vi "XY Scanning with Alazar.vi"() -> ()   [LabVIEW 2018]
uses:
  General/Controls/System Parameters.ctl
  General/Controls/Optical Parameters.ctl
  General/Controls/Vibratome Parameters.ctl
  General/Controls/Translation Stage Parameters.ctl
  Hardware Mfg/Thorlabs Translation Stages/Controls/Translation Stage Cluster.ctl
  General/Controls/Translation Stage Types.ctl
  General/Controls/Imaging Parameters.ctl
  General/Controls/Scan Direction.ctl
  Hardware Mfg/AlazarTech SDK/Controls/Clock Controls.ctl
  Hardware Mfg/AlazarTech SDK/Controls/Alazar Device ID.ctl
  Hardware Mfg/AlazarTech SDK/Controls/Channel Input Controls.ctl
  Hardware Mfg/AlazarTech SDK/Controls/General Trigger Settings.ctl
  Hardware Mfg/AlazarTech SDK/Controls/Trigger Engine Controls.ctl
  Hardware Mfg/AlazarTech SDK/Controls/Alazar Acquisition Settings.ctl
  General/actions/file type.ctl
  Hardware Mfg/AlazarTech SDK/Controls/Alazar Engine Actions.ctl
  General/Queue Manager Actions.ctl
  General/data manager action.ctl
  <vilib>/ErrorRing/Error Ring.xnode
panel:
  in  "file (use dialog)":path
  in  "File Type":T1
  in  "data action":enum16{"display", "save"}(ring)
  out "visulization time":dbl
  out "buffer enqueue time":dbl
  out "Image":T2(plugin-control)
  out "error out":errorcluster
  in  "stop":bool
  in  "Acq Settings":T3={"Window Type"=1, "Record Length"=1440, "Footer"=0, "Output Format"=11, "Offset"=0, "Records Per Buffer"=2048, "Records Count (Records/Acq)"=2147483647} {"Window Type" items=["DSP_WINDOW_NONE", "DSP_WINDOW_HANNING", "DSP_WINDOW_HAMMING", "DSP_WINDOW_BLACKMAN", "DSP_WINDOW_BLACKMAN_HARRIS", "DSP_WINDOW_BARTLETT"]; "Footer" items=["FOOTER_NONE", "FOOTER_NPT"]; "Output Format" items=["FLOAT_AMP2"=10, "FLOAT_LOG"=11]}
  in  "Trigger Settings":T6={"General Trigger Settings"={"Trigger Operation"=0, "Coupling ID"=2, "Range ID"=2, "Delay"=0, "Timeout Ticks"=0, "Mode"=0, "Parameter"=0}, "Trigger Engine 1"={"Trigger Engine"=0, "Source"=2, "Slope"=1, "Level"=140}, "Trigger Engine 2"={"Trigger Engine"=1, "Source"=3, "Slope"=1, "Level"=140}} {"General Trigger Settings"."Trigger Operation" items=["J", "K", "J OR K", "J AND K", "J XOR K", "J AND NOT K", "NOT J AND K"]; "General Trigger Settings"."Coupling ID" items=["AC"=1, "DC"=2]; "General Trigger Settings"."Range ID" items=["5 V", "1 V", "TTL"]; "Trigger Engine 1"."Trigger Engine" items=["J", "K"]; "Trigger Engine 1"."Source" items=["A", "B", "External", "Disable", "C", "D"]; "Trigger Engine 1"."Slope" items=["Positive"=1, "Negative"=2]; "Trigger Engine 2"."Trigger Engine" items=["J", "K"]; "Trigger Engine 2"."Source" items=["A", "B", "External", "Disable", "C", "D"]; "Trigger Engine 2"."Slope" items=["Positive"=1, "Negative"=2]}
  in  "Ch B Input Control":T7={"Channel"=2, "Coupling"=2, "Range"=10, "Impedance"=2} {"Channel" items=["A"=1, "B"=2, "C"=4, "D"=8]; "Coupling" items=["AC"=1, "DC"=2]; "Range" items=["20 mV"=1, "40 mV"=2, "50 mV"=3, "80 mV"=4, "100 mV"=5, "200 mV"=6, "400 mV"=7, "500 mV"=8, "800 mV"=9, "1 V"=10, "1.25 V"=33, "2 V"=11, "4 V"=12, "5 V"=13, "8 V"=14, "10 V"=15, "20 V"=16]; "Impedance" items=["1 MOhm"=1, "50 Ohm"=2, ""=0]}
  in  "Ch A Input Control":T7={"Channel"=1, "Coupling"=2, "Range"=10, "Impedance"=2} {"Channel" items=["A"=1, "B"=2, "C"=4, "D"=8]; "Coupling" items=["AC"=1, "DC"=2]; "Range" items=["20 mV"=1, "40 mV"=2, "50 mV"=3, "80 mV"=4, "100 mV"=5, "200 mV"=6, "400 mV"=7, "500 mV"=8, "800 mV"=9, "1 V"=10, "1.25 V"=33, "2 V"=11, "4 V"=12, "5 V"=13, "8 V"=14, "10 V"=15, "20 V"=16]; "Impedance" items=["1 MOhm"=1, "50 Ohm"=2, ""=0]}
  in  "Device ID":T8={"System ID"=1, "Board ID"=1}
  in  "Capture Clock":T9={"Sample Rate"=100, "Decimation"=0, "Source"=2, "Edge"=0} {"Edge" items=["Rising", "Falling"]; "Source" items=["Internal"=1, "Fast External"=2, "Medium External"=3, "Slow External"=4, "External AC"=5, "External DC"=6, "External 10MHz"=7]}
  in  "System Parameters":T10={"Optical Parameters"={"Obj. Focal Length [mm]"=45.0, "Scan Lens EFL[mm]"=60.0, "Tube Lens EFL[mm]"=180.0, "Galvo V Range (+/-)"=10.0, "Galvo Max Half Angle [Deg]"=19.0, "Max Galvo Range[%]"=0.0}, "Vibratome"={"Z Bottom [mm]"=0.0, "Pre Cut Dwell [s]"=0.0, "Blade Frequency [RPM]"=0, "Slice Speed [mm/s]"=0.0, "Post Cut Dwell [s]"=0.0, "Ramp Time [s]"=0.0, "Start X [mm]"=0.0, "Start Y [mm]"=0.0, "Slice Length [mm]"=0.0, "Slice Axis"=enum."Y Axis", "Controller VISA Ref"="COM4"}, "Table Stages"={"X Stage"={"Position"=0.0, "Is.Enabled?"=FALSE, "Is.Connected?"=FALSE, "Device SN"="45876539", "AccelerationMaximum"=0.0, "VelocityMaximum"=0.0, "Acceleration"=0.0, "Velocity"=0.0, "waitTimeout (ms)"=0, "Model"=enum."None", "Is.Homed?"=FALSE}, "Y Stage"={"Position"=0.0, "Is.Enabled?"=FALSE, "Is.Connected?"=FALSE, "Device SN"="45876539", "AccelerationMaximum"=0.0, "VelocityMaximum"=0.0, "Acceleration"=0.0, "Velocity"=0.0, "waitTimeout (ms)"=0, "Model"=enum."None", "Is.Homed?"=FALSE}, "Z Stage"={"Position"=0.0, "Is.Enabled?"=FALSE, "Is.Connected?"=FALSE, "Device SN"="45876539", "AccelerationMaximum"=0.0, "VelocityMaximum"=0.0, "Acceleration"=0.0, "Velocity"=0.0, "waitTimeout (ms)"=0, "Model"=enum."None", "Is.Homed?"=FALSE}}, "Imaging Parameter"={"Raster Scan Direction"=enum."Uni Directional", "Pixel Dwell Time [Clock Cycles]"=1, "Flyback Time [Clock Cycles]"=150, "XY Center [um]"={"X"=1.0, "Y"=1.0}, "Pixel Step Size [um]"=4.0, "XY Image Size"=enum."2048 x 2048", "Custom"=FALSE, "Custom Size"={"X"=10, "Y"=10}, "Line Averages"=1}} {"Imaging Parameter"."Line Averages" min=1 max=30 step=1; "Imaging Parameter"."Flyback Time [Clock Cycles]" max=1000 step=1; "Imaging Parameter"."Pixel Step Size [um]" min=0.0 max=10.0 step=0.01; "Imaging Parameter"."Custom Size"."Y" min=1 max=30 step=1; "Imaging Parameter"."Custom Size"."X" min=1 max=30 step=1; "Imaging Parameter"."XY Center [um]"."Y" min=1.0 max=30.0 step=1.0; "Imaging Parameter"."XY Center [um]"."X" min=1.0 max=30.0 step=1.0; "Imaging Parameter"."Pixel Dwell Time [Clock Cycles]" max=10 step=1}
  in  "Galvo HW Parameters":T18={"Analog Out Channel"="GalvoCtrl/ao0,GalvoCtrl/ao1", "Min Voltage"=-10.0, "Max Voltage"=10.0, "Pixel Clock Source"="/GalvoCtrl/PFI0", "Sample Rate"=1000.0, "Line Clock Out Ch"="GalvoCtrl/port0/line0"}
  # "X"
  # "X"
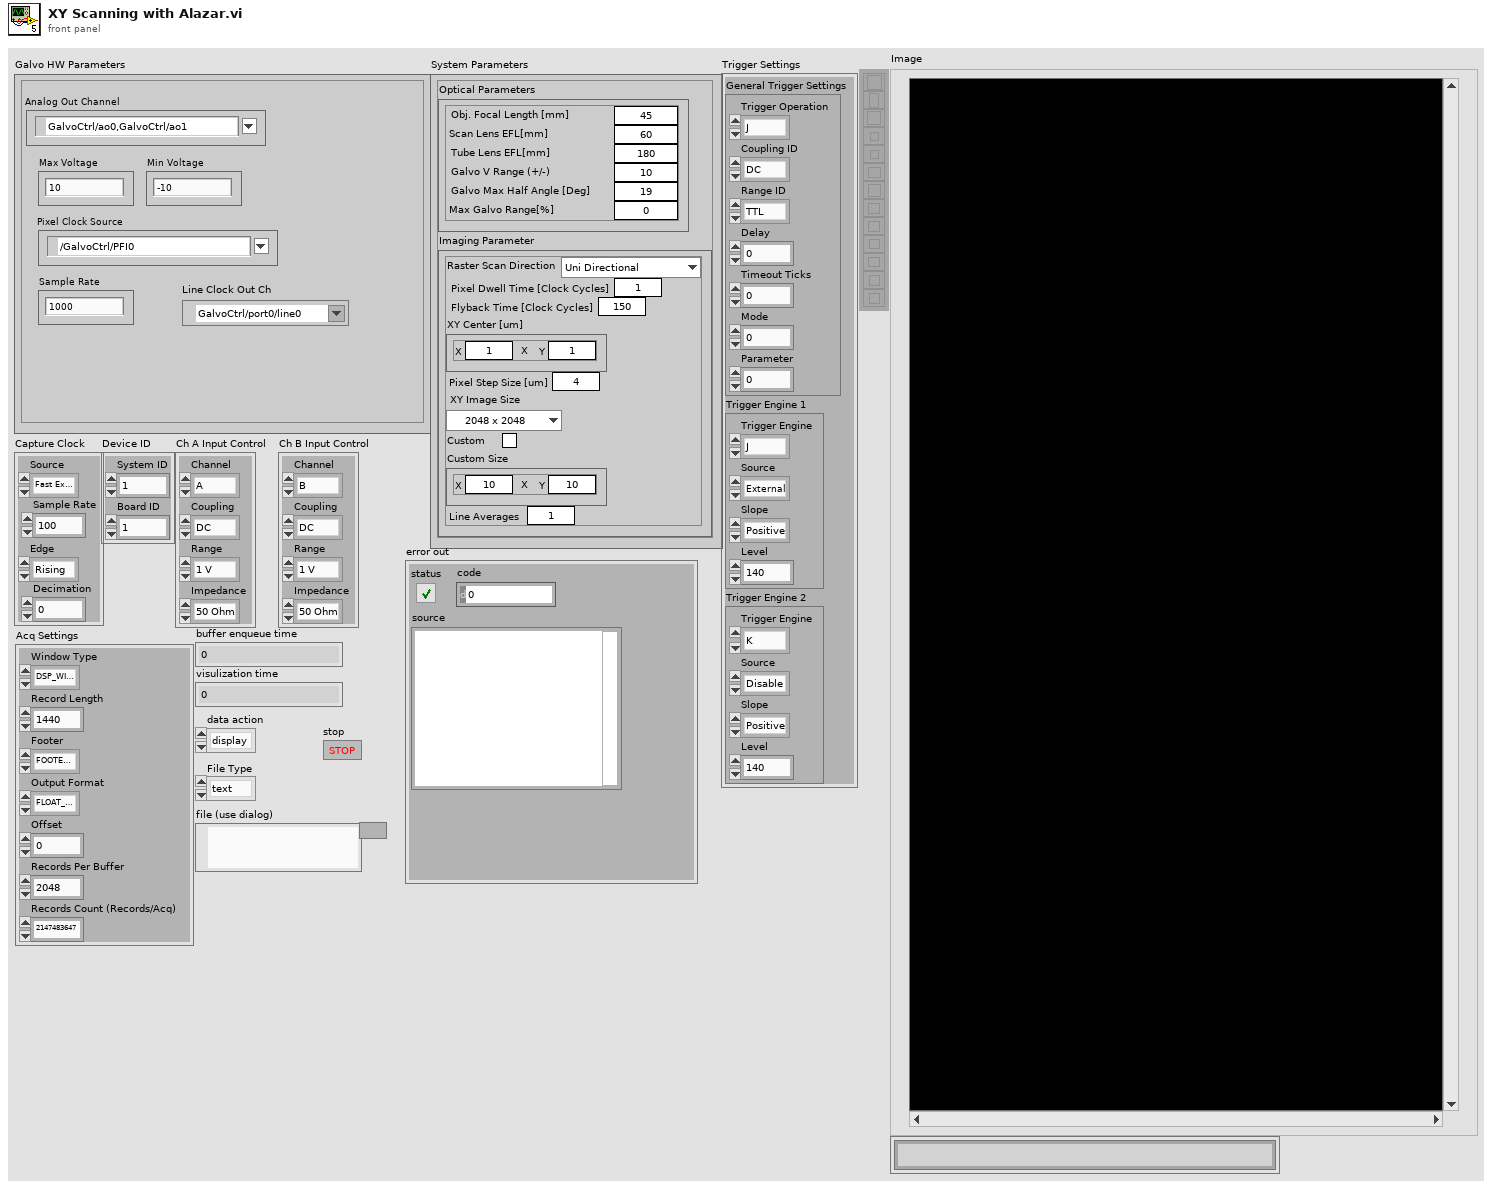
[diagram p1: front panel]
types:
  T1 = typedef "file type.ctl" = enum16{"text", "image", "binary"}
  T2 = typedef "IMAQ Image.ctl" = refnum<image>
  T3 = typedef "Alazar Acquisition Settings.ctl" = cluster{"Window Type":u32, "Record Length":u32, "Footer":u32, "Output Format":u32, "Offset":u32, "Records Per Buffer":u32, "Records Count (Records/Acq)":u32}
  T4 = typedef "General Trigger Settings.ctl" = cluster{"Trigger Operation":u32, "Coupling ID":u32, "Range ID":u32, "Delay":u32, "Timeout Ticks":u32, "Mode":u32, "Parameter":u32}
  T5 = typedef "Trigger Engine Controls.ctl" = cluster{"Trigger Engine":u32, "Source":u32, "Slope":u32, "Level":u32}
  T6 = cluster{"General Trigger Settings":T4, "Trigger Engine 1":T5, "Trigger Engine 2":T5}
  T7 = typedef "Channel Input Controls.ctl" = cluster{"Channel":u8, "Coupling":u32, "Range":u32, "Impedance":u32}
  T8 = typedef "Alazar Device ID.ctl" = cluster{"System ID":u32, "Board ID":u32}
  T9 = typedef "Clock Controls.ctl" = cluster{"Sample Rate":u32, "Decimation":u32, "Source":u32, "Edge":u32}
  T10 = typedef "System Parameters.ctl" = cluster{"Optical Parameters":T11, "Vibratome":T12, "Table Stages":T13, "Imaging Parameter":T16}
  T11 = typedef "Optical Parameters.ctl" = cluster{"Obj. Focal Length [mm]":dbl, "Scan Lens EFL[mm]":dbl, "Tube Lens EFL[mm]":dbl, "Galvo V Range (+/-)":dbl, "Galvo Max Half Angle [Deg]":dbl, "Max Galvo Range[%]":dbl}
  T12 = typedef "Vibratome Parameters.ctl" = cluster{"Z Bottom [mm]":dbl, "Pre Cut Dwell [s]":dbl, "Blade Frequency [RPM]":u16, "Slice Speed [mm/s]":dbl, "Post Cut Dwell [s]":dbl, "Ramp Time [s]":dbl, "Start X [mm]":dbl, "Start Y [mm]":dbl, "Slice Length [mm]":dbl, "Slice Axis":enum16{"X Axis", "Y Axis", "Z Axis"}, "Controller VISA Ref":refnum<visa-resource-name>}
  T13 = typedef "Translation Stage Parameters.ctl" = cluster{"X Stage":T14, "Y Stage":T14, "Z Stage":T14}
  T14 = typedef "Translation Stage Cluster.ctl" = cluster{"Position":dbl, "Is.Enabled?":bool, "Is.Connected?":bool, "Device SN":string, "AccelerationMaximum":dbl, "VelocityMaximum":dbl, "Acceleration":dbl, "Velocity":dbl, "waitTimeout (ms)":i32, "Model":T15, "Is.Homed?":bool}
  T15 = typedef "Translation Stage Types.ctl" = enum16{"None", "Thorlabs LTS", "Thorlabs MLJ"}
  T16 = typedef "Imaging Parameters.ctl" = cluster{"Raster Scan Direction":T17, "Pixel Dwell Time [Clock Cycles]":u16, "Flyback Time [Clock Cycles]":u16, "XY Center [um]":cluster{"X":dbl, "Y":dbl}, "Pixel Step Size [um]":dbl, "XY Image Size":enum16{"32 x 32", "64 x 64", "128 x 128", "256 x 256", "512 x 512", "1024 x 1024", "2048 x 2048"}, "Custom":bool, "Custom Size":cluster{"X":u16, "Y":u16}, "Line Averages":u8}
  T17 = typedef "Scan Direction.ctl" = enum16{"Uni Directional", "Bi Directional", "None"}
  T18 = cluster{"Analog Out Channel":tag, "Min Voltage":dbl, "Max Voltage":dbl, "Pixel Clock Source":tag, "Sample Rate":dbl, "Line Clock Out Ch":tag}
  T19 = typedef "Queue Manager Actions.ctl" = enum16{"Init", "Enqueue", "Enqueue All", "Preview Queue", "Dequeue", "Get Status", "Flush Queue", "Flush All Queues", "Release All Queues", "Release Queue", "Enqueue at Opposite End"}
  T20 = typedef "Alazar Engine Actions.ctl" = enum16{"Init", "Config Clock", "Config Ch", "Config Trig", "Config Acq.", "Acquire", "UnInit"}
  T21 = enum16{"Init", "Calc & Write Scan Pattern", "Start Galvo Task", "Is Task Done?", "Stop Galvo", "Uninit"}
  T22 = typedef "data manager action.ctl" = enum16{"", "open file", "close file", "display non IMAQ", "display", "save"}
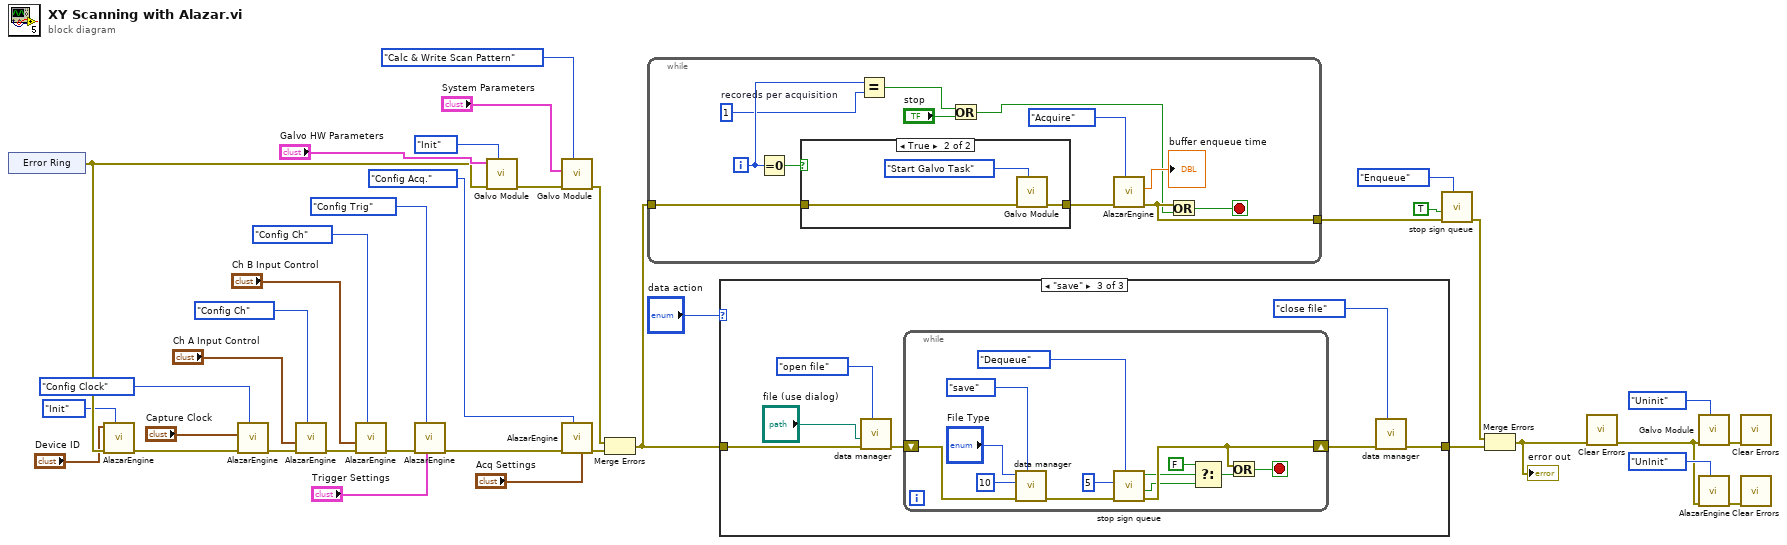
[diagram p0: block diagram]
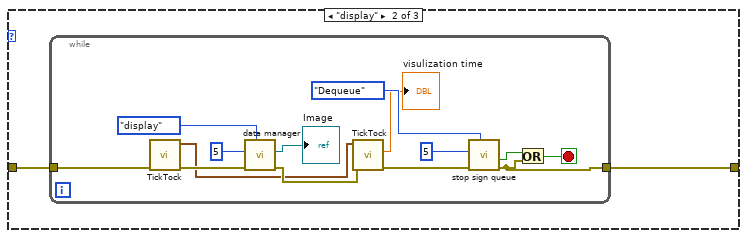
[diagram p3: hidden frame]
diagram:
  n1 = xnode "Error Ring"() -> ("error out"=w29:errorcluster)
  n2 = call "AlazarEngine.vi"("Action"=Alazar_Engine_Actions."Init", "error in (no error)"=w29, "Device ID"="Device ID") -> ("error out"=w32:errorcluster)  [unwired: 7 in, 1 out]
  n3 = call "AlazarEngine.vi"("Action"=Alazar_Engine_Actions."Config Clock", "error in (no error)"=w32, "Capture Clock"="Capture Clock") -> ("error out"=w31:errorcluster)  [unwired: 7 in, 1 out]
  n4 = call "AlazarEngine.vi"("Action"=Alazar_Engine_Actions."Config Ch", "error in (no error)"=w31, "Ch Input Control"="Ch A Input Control") -> ("error out"=w30:errorcluster)  [unwired: 7 in, 1 out]
  n5 = call "AlazarEngine.vi"("Action"=Alazar_Engine_Actions."Config Ch", "error in (no error)"=w30, "Ch Input Control"="Ch B Input Control") -> ("error out"=w20:errorcluster)  [unwired: 7 in, 1 out]
  n6 = call "AlazarEngine.vi"("Trigger Settings"="Trigger Settings", "Action"=Alazar_Engine_Actions."Config Trig", "error in (no error)"=w20) -> ("error out"=w17:errorcluster)  [unwired: 7 in, 1 out]
  n7 = call "Galvo Module.vi"("Action"=T21."Init", "error in (no error)"=w29, "Galvo HW Parameters"="Galvo HW Parameters") -> ("error out"=w36:errorcluster)  [unwired: 7 in, 1 out]
  n8 = call "Galvo Module.vi"("Action"=T21."Calc & Write Scan Pattern", "error in (no error)"=w36, "System Parameters"="System Parameters") -> ("error out"=w35:errorcluster)  [unwired: 7 in, 1 out]
  n9 = call "AlazarEngine.vi"("Acq Settings"="Acq Settings", "Action"=Alazar_Engine_Actions."Config Acq.", "error in (no error)"=w17) -> ("error out"=w14:errorcluster)  [unwired: 7 in, 1 out]
  n10 = Merge Errors(w35, w14) -> (w8:errorcluster)
  n11 = while {
    tunnel: w8 -> [w50]
    tunnel: [w46] -> w5
    i -> [w43]
    stop <- w45 stop-if-true
    w42 = 1  # recoreds per acquisition
    n12 = Equal To 0?(x=w43) -> (x = 0?=w49:bool)
    n13 = case shown="True" w49 {
      tunnel: w50 -> [w51 w54]
      tunnel: [w51 w52] -> w48
      frame False {
      }
      frame True {
        n14 = call "Galvo Module.vi"("Action"=T21."Start Galvo Task", "error in (no error)"=w54) -> ("error out"=w52:errorcluster)  [unwired: 8 in, 1 out]
      }
    }
    n15 = Equal?(x=w43, y=w42) -> (x = y?=w41:bool)
    n16 = Or(x=w41, y="stop") -> (x .or. y?=w39:bool)
    n17 = call "AlazarEngine.vi"("Action"=Alazar_Engine_Actions."Acquire", "error in (no error)"=w48) -> ("error out"=w46:errorcluster, "dt"=→"buffer enqueue time":dbl)  [unwired: 8 in]
    n18 = Or(x=w46, y=w39) -> (x .or. y?=w45:bool)
  }
  n19 = case shown="\"save\"" "data action" {
    tunnel: w8 -> [w55 w57 w76]
    tunnel: [w55 w56 w73] -> w7
    frame Default {
    }
    frame "display" {
      n20 = while {
        tunnel: w57 -> [w69]
        tunnel: [w70] -> w56
        stop <- w71 stop-if-true
        n21 = call "TickTock.vi"("Error In"=w69) -> ("Error Out"=w63:errorcluster, "Current Time (Out)"=w60:timestamp)  [unwired: 8 in, 1 out]
        n22 = call "data manager.vi"("action"=data_manager_action."display", "error in (no error)"=w63, "timeout in ms (-1)"=5) -> ("error out"=w62:errorcluster, "Image"=→"Image":T2)  [unwired: 6 in, 1 out]
        n23 = call "TickTock.vi"("Error In"=w62, "Current Time (In)"=w60) -> ("Error Out"=w61:errorcluster, "dt"=→"visulization time":dbl)  [unwired: 7 in, 1 out]
        n24 = call "stop sign queue.vi"("Action"=Queue_Manager_Actions."Dequeue", "error in (no error)"=w61, "time out"=5) -> ("error out"=w70:errorcluster, "stop out"=w65:bool)  [unwired: 5 in, 2 out]
        n25 = Or(x=w65, y=w70) -> (x .or. y?=w71:bool)
      }
    }
    frame "save" {
      n26 = call "data manager.vi"("action"=data_manager_action."open file", "error in (no error)"=w76, "file (use dialog)"="file (use dialog)") -> ("error out"=w75:errorcluster)  [unwired: 6 in, 2 out]
      n27 = while {
        shift-right: [w85] -> w74
        shift-left: w75 -> [w90]
        stop <- w88 stop-if-true
        n28 = call "data manager.vi"("action"=data_manager_action."save", "error in (no error)"=w90, "timeout in ms (-1)"=10, "File Type"="File Type") -> ("error out"=w86:errorcluster)  [unwired: 5 in, 2 out]
        n29 = call "stop sign queue.vi"("Action"=Queue_Manager_Actions."Dequeue", "error in (no error)"=w86, "time out"=5) -> ("error out"=w85:errorcluster, "stop out"=w80:bool, "timed out?"=w82:bool)  [unwired: 5 in, 1 out]
        n30 = Select(t=FALSE, s=w82, f=w80) -> (s? t:f=w79:bool)
        n31 = Or(x=w85, y=w79) -> (x .or. y?=w88:bool)
      }
      n32 = call "data manager.vi"("action"=data_manager_action."close file", "error in (no error)"=w74) -> ("error out"=w73:errorcluster)  [unwired: 7 in, 2 out]
    }
  }
  n33 = call "stop sign queue.vi"("Action"=Queue_Manager_Actions."Enqueue", "error in (no error)"=w5, "stop in"=TRUE) -> ("error out"=w4:errorcluster)  [unwired: 5 in, 3 out]
  n34 = Merge Errors(w4, w7) -> (w6:errorcluster)
  "error out" <- w6
  n35 = call <vilib>:"Clear Errors.vi"("error in (no error)"=w6) -> ("error out"=w11:errorcluster)  [unwired: 5 in, 1 out]
  n36 = call "Galvo Module.vi"("Action"=T21."Uninit", "error in (no error)"=w11) -> ("error out"=w10:errorcluster)  [unwired: 8 in, 1 out]
  n37 = call "AlazarEngine.vi"("Action"=Alazar_Engine_Actions."UnInit", "error in (no error)"=w11) -> ("error out"=w9:errorcluster)  [unwired: 8 in, 1 out]
  n38 = call <vilib>:"Clear Errors.vi"("error in (no error)"=w10) -> ()  [unwired: 5 in, 2 out]
  n39 = call <vilib>:"Clear Errors.vi"("error in (no error)"=w9) -> ()  [unwired: 5 in, 2 out]
